vi "LogErrInfo.vi"(10 "location info":string, 11 "error in (no error)":errorcluster) -> (3 "error out":errorcluster)   [LabVIEW 2020]
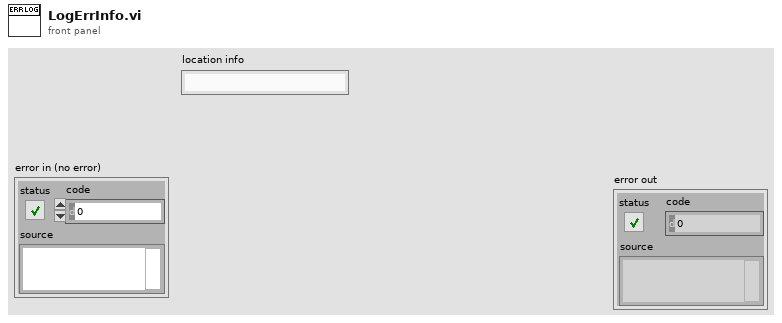
[diagram p1: front panel]
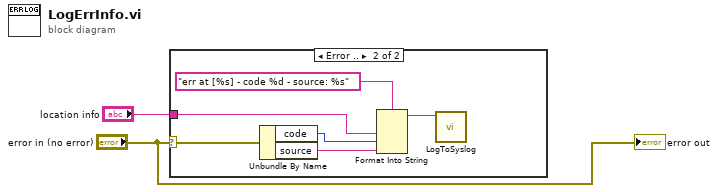
[diagram p0: block diagram]
diagram:
  n1 = case shown="Error .." "error in (no error)" {
    selector: "error in (no error)" -> [_ w8]
    tunnel: "location info" -> [_ w4]
    frame No Error {
    }
    frame Error {
      n2 = Unbundle By Name(w8) -> ("code"=w7:i32, "source"=w6:string)
      n3 = Format Into String(format string="err at [%s] - code %d - source: %s", w4, w7, w6) -> (resulting string=w3:string)  [unwired: 2 in, 1 out]
      n4 = call "LogToSyslog.vi"("message"=w3) -> ()  [unwired: 9 in, 2 out]
    }
  }
  "error out" <- "error in (no error)"
